vi "DeQueue&VTD.vi"(0 "ModuleAdmin In":refnum<class "ModuleAdmin.lvclass">, 2 "DeQueue Type (DeQueue)":T2, 5 "timeout in ms (100)":i32=50, 11 "Error In":errorcluster, 13 "QueueArrayEntry(QMH)":T1) -> (4 "ModuleAdmin Out":refnum<class "ModuleAdmin.lvclass">, 6 "Message":string, 8 "Message Data":variant, 10 "Class":refnum<class "AnalysisPluginsBase.lvclass">, 14 "Timed Out":bool, 15 "Error Out":errorcluster)   [LabVIEW 2018, in "AnalysisModule.lvlib"]
uses:
  AnalysisModule.lvlib
  <userlib>/NIST/ModuleAdminLib/ModuleAdmin/ModuleAdmin.lvclass
  <userlib>/NIST/ModuleAdminLib/ModuleAdmin/TypeDefinitions/DeQueueType.ctl
  <userlib>/NIST/ModuleAdminLib/ModuleAdmin/TypeDefinitions/QueueEntry.ctl
  AnalysisPlugins/AnalysisPluginBaseClass/AnalysisPluginsBase.lvclass
  clAnalysisMsg.ctl
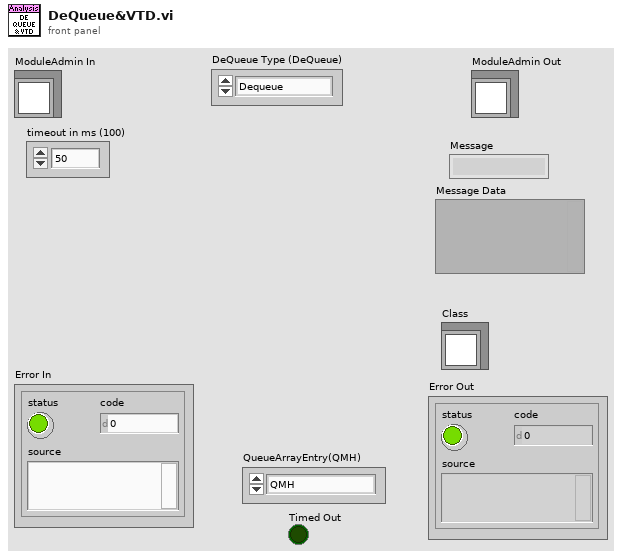
[diagram p1: front panel]
types:
  T1 = typedef "ModuleAdmin.lvlib/ModuleAdmin.lvclass/QueueEntry.ctl" = enum16{"QMH", "Class Data", "Data Loop", "Queue 4", "Queue 5", "Queue 6", "Queue 7", "Queue 8", "Queue 9", "Queue 10"}
  T2 = typedef "ModuleAdmin.lvlib/ModuleAdmin.lvclass/DeQueueType.ctl" = enum16{"Dequeue", "PreviewQueue"}
  T3 = typedef "AnalysisModule.lvlib/clAnalysisMsg.ctl" = cluster{"Class":refnum<class "AnalysisPluginsBase.lvclass">, "Message":string, "Message Data":variant}
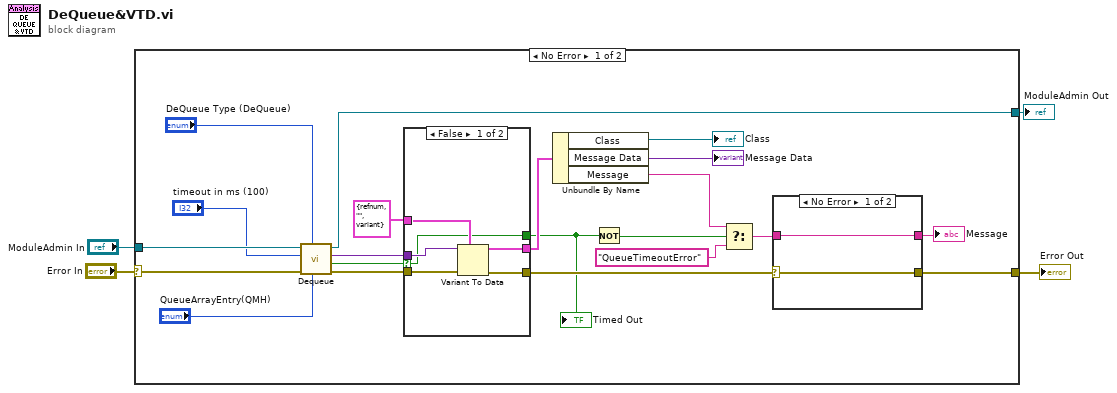
[diagram p0: block diagram]
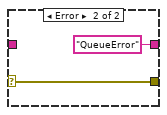
[diagram p2: hidden frame]
diagram:
  n1 = case shown="No Error" "Error In" {
    selector: "Error In" -> [w23 w40]
    tunnel: "ModuleAdmin In" -> [w24 w39]
    tunnel: [w17 w39] -> w2
    tunnel: [w6 w40] -> w1
    frame No Error {
      n2 = call <userlib>:"Dequeue.vi"("QueueArrayEntry (QMH)"="QueueArrayEntry(QMH)", "DeQueue Type (DeQueue)"="DeQueue Type (DeQueue)", "error in (no error)"=w23, "timeout in ms (100)"="timeout in ms (100)", "ModuleAdmin In"=w24) -> ("error out"=w19:errorcluster, "timed out?"=w20:bool, "Element"=w18:variant, "ModuleAdmin Out"=w17:refnum<class "ModuleAdmin.lvclass">)  [unwired: 3 in]
      n3 = case shown="False" w20 {
        selector: w20 -> [w30 w36]
        tunnel: w19 -> [w35 w37]
        tunnel: w18 -> [w34 _]
        tunnel: T3 {"Class"=refnum, "Message"="", "Message Data"=variant} ("clAnalysisMsg") -> [w33 w38]
        tunnel: [w32 w38] -> w15
        tunnel: [w31 w37] -> w13
        tunnel: [w30 w36] -> w9
        frame False {
          n4 = Variant To Data(error in=w35, type=w33, Variant=w34) -> (data=w32:T3, error out=w31:errorcluster)
        }
        frame True {
          # "If Timeout, there will be no data"
        }
      }
      "Timed Out" <- w9
      n5 = Unbundle By Name(w15) -> ("Class"=→"Class":refnum<class "AnalysisPluginsBase.lvclass">, "Message Data"=→"Message Data":variant, "Message"=w11:string)
      n6 = Not(x=w9) -> (.not. x?=w10:bool)
      n7 = Select(t=w11, s=w10, f="QueueTimeoutError") -> (s? t:f=w8:string)
      n8 = case shown="No Error" w13 {
        selector: w13 -> [w26 w28]
        tunnel: w8 -> [w27 _]
        tunnel: [w27 "QueueError" ("Message")] -> w7
        tunnel: [w26 w28] -> w6
        frame No Error {
        }
        frame Error {
        }
      }
      "Message" <- w7
    }
    frame Error {
    }
  }
  "ModuleAdmin Out" <- w2
  "Error Out" <- w1
